vi "PPT_configure.vi"() -> ()   [LabVIEW 2010]
panel:
  in  "Port Name":string
  out "Read":string
  out "?":string
  in  "Integration Number":i16=70 min=0 max=120
  in  "Rate(F) or interval(T)":bool=TRUE
  in  "Display Units":u16(ring)=1 items=["Atmospheres", "Bar", "Centimetres Water @4C", "Feet water @4C", "Inches of Mercury @0C", "Inches Water @4C", "Kg/cm^2", "KPa", "Millibar", "Millimeters Mercury @0C (Torr)", "MPa", "Metres Water @4C", "PSI", "User defined", "Logic common value", "Percent of Full Scale"]
  in  "New Address":u8=50 max=89
  in  "Old Address":u8 max=89
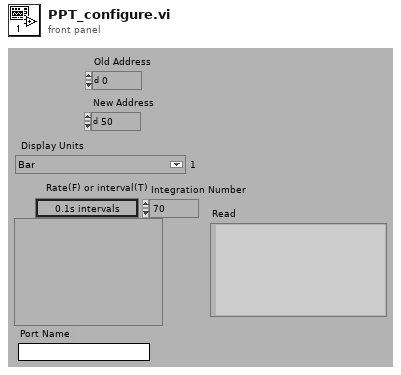
[diagram p1: front panel]
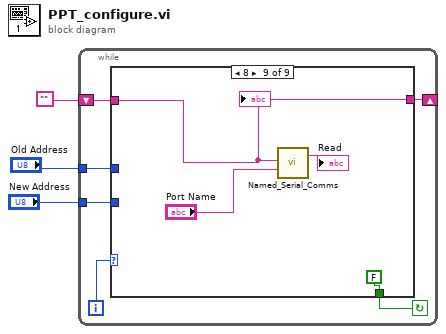
[diagram p0: block diagram]
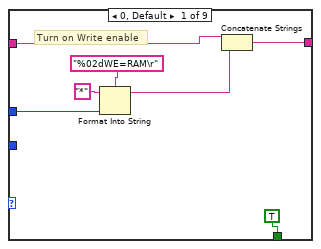
[diagram p2: hidden frame]
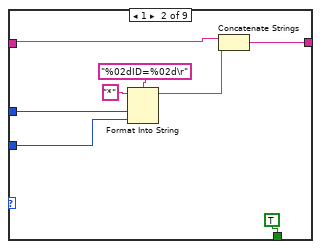
[diagram p3: hidden frame]
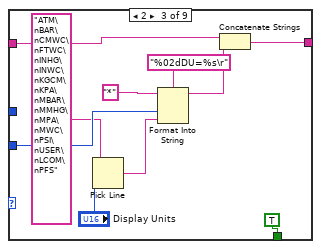
[diagram p4: hidden frame]
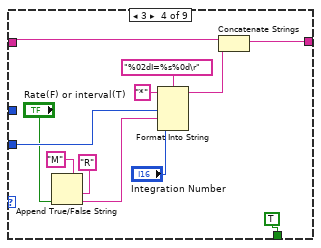
[diagram p5: hidden frame]
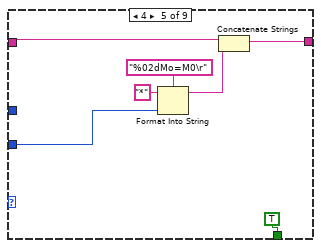
[diagram p6: hidden frame]
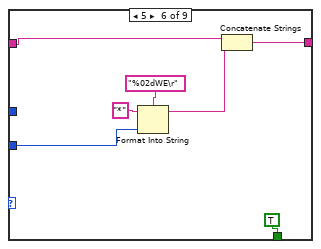
[diagram p7: hidden frame]
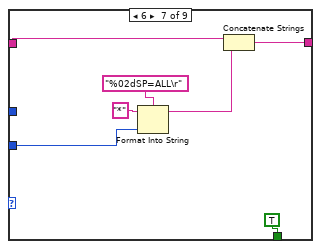
[diagram p8: hidden frame]
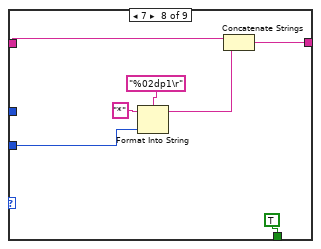
[diagram p9: hidden frame]
diagram:
  n1 = while {
    shift-left: "" -> [w4]
    shift-right: [w5] -> _
    tunnel: "New Address" -> [w8]
    tunnel: "Old Address" -> [w9]
    i -> [w7]
    stop <- w6 continue-if-true
    n2 = case shown="8" w7 {
      tunnel: w9 -> [w14 w22 _ _ _ _ _ _ _]
      tunnel: w8 -> [_ w21 w32 w44 w51 w58 w65 w72 _]
      tunnel: [TRUE TRUE TRUE TRUE TRUE TRUE TRUE TRUE FALSE] -> w6
      tunnel: [w12 w17 w25 w35 w47 w54 w63 w70 w77] -> w5
      tunnel: w4 -> [w11 w19 w27 w36 w48 w56 w61 w68 w77]
      frame 0, Default {
        # "Turn on Write enable"
        n3 = Format Into String(format string="%02dWE=RAM\r", initial string="*", w14) -> (resulting string=w10:string)  [unwired: 1 in, 1 out]
        n4 = Concatenate Strings(w11, w10) -> (w12:string)
      }
      frame 1 {
        n5 = Format Into String(format string="%02dID=%02d\r", initial string="*", w22, w21) -> (resulting string=w18:string)  [unwired: 1 in, 1 out]
        n6 = Concatenate Strings(w19, w18) -> (w17:string)
      }
      frame 2 {
        n7 = Pick Line(multi-line string="ATM\nBAR\nCMWC\nFTWC\nINHG\nINWC\nKGCM\nKPA\nMBAR\nMMHG\nMPA\nMWC\nPSI\nUSER\nLCOM\nPFS", line index="Display Units") -> (output string=w29:string)  [unwired: 1 in]
        n8 = Format Into String(format string="%02dDU=%s\r", initial string="*", w32, w29) -> (resulting string=w26:string)  [unwired: 1 in, 1 out]
        n9 = Concatenate Strings(w27, w26) -> (w25:string)
      }
      frame 3 {
        n10 = Append True/False String(1:"Rate(F) or interval(T)", 2:"R" ("false string"), 3:"M" ("true string")) -> (0:w39:string)  [unwired: 1 in]
        n11 = Format Into String(format string="%02dI=%s%0d\r", initial string="*", w44, w39, "Integration Number") -> (resulting string=w43:string)  [unwired: 1 in, 1 out]
        n12 = Concatenate Strings(w36, w43) -> (w35:string)
      }
      frame 4 {
        n13 = Format Into String(format string="%02dMo=M0\r", initial string="*", w51) -> (resulting string=w50:string)  [unwired: 1 in, 1 out]
        n14 = Concatenate Strings(w48, w50) -> (w47:string)
      }
      frame 5 {
        n15 = Format Into String(format string="%02dWE\r", initial string="*", w58) -> (resulting string=w55:string)  [unwired: 1 in, 1 out]
        n16 = Concatenate Strings(w56, w55) -> (w54:string)
      }
      frame 6 {
        n17 = Format Into String(format string="%02dSP=ALL\r", initial string="*", w65) -> (resulting string=w62:string)  [unwired: 1 in, 1 out]
        n18 = Concatenate Strings(w61, w62) -> (w63:string)
      }
      frame 7 {
        n19 = Format Into String(format string="%02dp1\r", initial string="*", w72) -> (resulting string=w69:string)  [unwired: 1 in, 1 out]
        n20 = Concatenate Strings(w68, w69) -> (w70:string)
      }
      frame 8 {
        n21 = call "Named_Serial_Comms.vi"("Write String"=w77, "Port Name"="Port Name") -> ("Read"=→"Read":string)  [unwired: 10 in, 3 out]
        "?" <- w77
      }
    }
  }
